vi "arithmetic_functions.vi"() -> ()   [LabVIEW 2018]
panel:
  in  "y":dbl
  in  "x":dbl
  out "x+y":dbl
  out "x*y":dbl
  out "x-y":dbl
  out "x/y":dbl
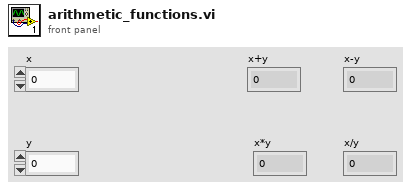
[diagram p1: front panel]
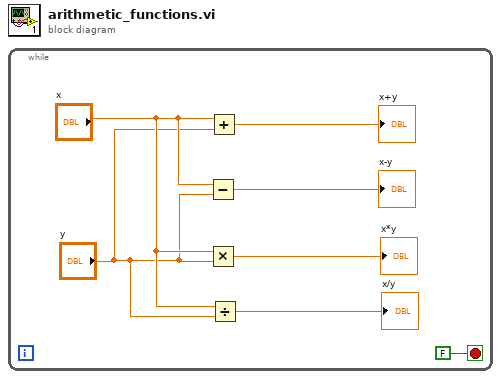
[diagram p0: block diagram]
diagram:
  n1 = while {
    stop <- FALSE stop-if-true
    n2 = Subtract(x="x", y="y") -> (x-y=→"x-y":dbl)
    n3 = Multiply(x="x", y="y") -> (x*y=→"x*y":dbl)
    n4 = Add(x="x", y="y") -> (x+y=→"x+y":dbl)
    n5 = Divide(x="x", y="y") -> (x/y=→"x/y":dbl)
  }
